vi "ReadDefaultConfig.vi"(8 "path":path, 11 "File":string) -> (0 "error out":errorcluster, 2 "path":path, 3 "config":T1={"Bead locations"=[{"X"=0, "Y"=0}], "ROI"=80, "Experiment base path"=path "", "Image output subdir"="images", "Output mode"=enum."Track", "Traces output subdir"="traces", "QTrk Settings"={"Image width"=100, "Image height"=100, "Number of threads (CPU based)"=-1, "CUDA Device"=-2, "COM Background correction factor"=0.0, "ZLUT MinRadius"=2.0, "ZLUT Radial sample density"=2.0, "ZLUT Angular sample density"=0.7, "ZLUT ROI Coverage"=1.0, "QI Iterations"=5, "QI MinRadius"=2.0, "QI Radial sample density"=2.0, "QI Angular sample density"=0.7, "QI ROI Coverage"=1.0, "QI Angular Step \nIteration Factor"=1.0, "XCOR Profile Length"=1, "XCOR Profile Width"=128, "XCOR Iterations"=32, "Gaussian 2D Fit Iterations"=2, "Gaussian 2D Sigma (pixels)"=3.0, "Downsample"=0}, "Tracking Config"={"Number of steps"=100, "ZLUT stepsize (um)"=0.05, "Z correction factor"=0.88, "Start piezo Z (um)"=0.0, "Pixel size (nm)"=146.0, "2D Localization Type"=enum."Quadrant Interpolation", "Z Command (None)"=enum."ComputeZ", "Z Piezo scale"=FALSE, "ZLUT Building\nimages per frame"=1, "ZLUT Bias correction planes"=1}, "Experiment Name"="test", "Program"={"Commands"=[], "Motor Axis accuracy conditions"={"Magnet Z"=0.0, "Magnet rotation"=0.0, "Camera"={"X"=0.0, "Y"=0.0}, "Piezo XY"={"X"=0.0, "Y"=0.0}, "Piezo Z"=0.0}, "Axis flags"={"Magnet Z"=FALSE, "Magnet rotation"=FALSE, "Camera"={"X"=FALSE, "Y"=FALSE}, "Piezo XY"={"X"=FALSE, "Y"=FALSE}, "Piezo Z"=FALSE}}, "ZLUT"=[], "Camera settings"={"Framerate (Hz)"=60, "Exposure time (us)"=5000, "Image size"={"Width"=1280, "Height"=1024}, "Number of buffers"=30}, "Experiment Script"="", "Max frames in memory"=100000, "Save traces as binary"=FALSE, "Pixel Calibration Gain Image"="camera_calib_gain.bin", "Pixel Calibration Offset Image"="camera_calib_offset.bin", "Use pixel calibration images"=FALSE, "Internal camera settings"="", "Trace write interval"=100, "ExperimentComment"=""} {"QTrk Settings"."QI ROI Coverage" format="%_2g"; "QTrk Settings"."QI MinRadius" format="%.2f"; "QTrk Settings"."QI Angular sample density" format="%.3f"; "QTrk Settings"."QI Radial sample density" format="%.2f"; "QTrk Settings"."ZLUT Radial sample density" format="%.2f"; "QTrk Settings"."ZLUT MinRadius" format="%.2f"})   [LabVIEW 2011]
uses:
  Main/Typedefs/MeasureConfigType.ctl
  Main/Typedefs/MeasureConfigOutputMode.ctl
  qtrk/QTrkLVBinding/QTrkSettings.ctl
  Main/Typedefs/TrackingConfigType.ctl
  qtrk/QTrkLVBinding/QTrkLocalizationType.ctl
  qtrk/QTrkLVBinding/QTrkZCommandType.ctl
  Main/ExperimentProgram/ExperimentProgramType.ctl
  Main/ExperimentProgram/ExProgCommandType.ctl
  Main/ExperimentProgram/ExProgCommandEnumType.ctl
  Main/Motors/MotorAxisEnum.ctl
  Main/Motors/MotorPosType.ctl
  Main/Typedefs/XYf.ctl
  Main/Motors/MotorPosFlagsType.ctl
  Main/Camera/GenericCameraConfigType.ctl
  Main/GlobalVariables.vi
  <vilib>/regexp/Match Regular Expression.xnode
panel:
  # "(used for commands with string parameters)"
  # "-2: Use all devices\n-1: Use best device"
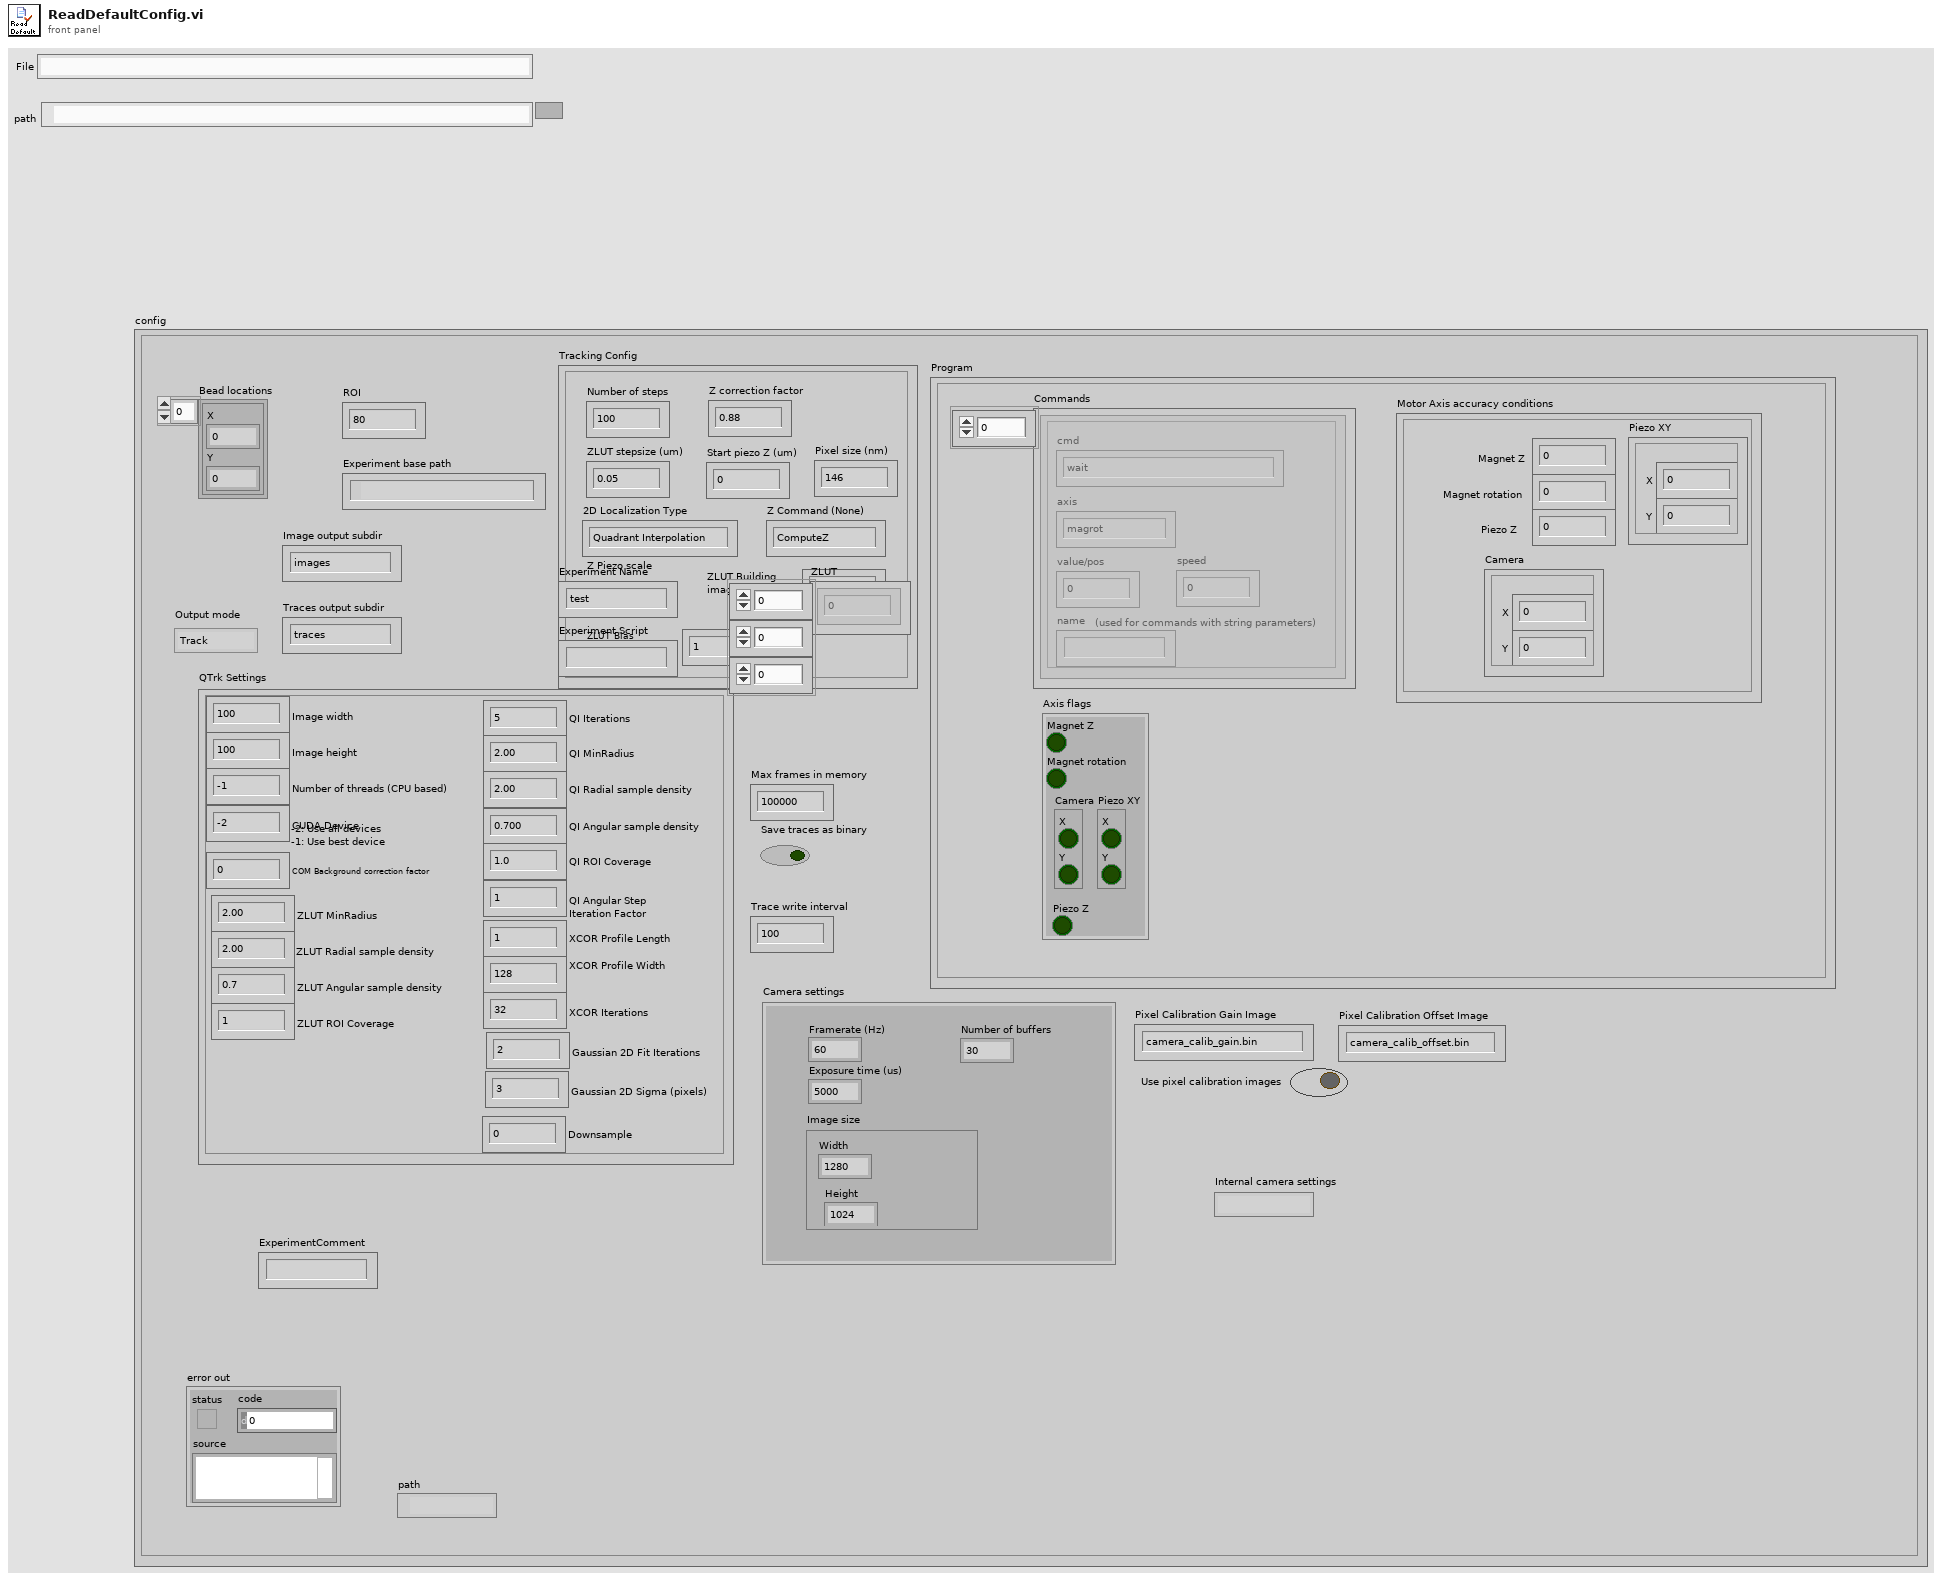
[diagram p1: front panel]
types:
  T1 = typedef "MeasureConfigType.ctl" = cluster{"Bead locations":cluster{"X":i32, "Y":i32}[], "ROI":i32, "Experiment base path":path, "Image output subdir":string, "Output mode":T2, "Traces output subdir":string, "QTrk Settings":T3, "Tracking Config":T4, "Experiment Name":string, "Program":T7, "ZLUT":sgl[][][], "Camera settings":T14, "Experiment Script":string, "Max frames in memory":i32, "Save traces as binary":bool, "Pixel Calibration Gain Image":string, "Pixel Calibration Offset Image":string, "Use pixel calibration images":bool, "Internal camera settings":string, "Trace write interval":i32, "ExperimentComment":string}
  T2 = typedef "MeasureConfigOutputMode.ctl" = enum16{"None", "Track", "SaveImages"}
  T3 = typedef "QTrkSettings.ctl" = cluster{"Image width":i32, "Image height":i32, "Number of threads (CPU based)":i32, "CUDA Device":i32, "COM Background correction factor":sgl, "ZLUT MinRadius":sgl, "ZLUT Radial sample density":sgl, "ZLUT Angular sample density":sgl, "ZLUT ROI Coverage":sgl, "QI Iterations":i32, "QI MinRadius":sgl, "QI Radial sample density":sgl, "QI Angular sample density":sgl, "QI ROI Coverage":sgl, "QI Angular Step \nIteration Factor":sgl, "XCOR Profile Length":i32, "XCOR Profile Width":i32, "XCOR Iterations":i32, "Gaussian 2D Fit Iterations":i32, "Gaussian 2D Sigma (pixels)":sgl, "Downsample":i32}
  T4 = typedef "TrackingConfigType.ctl" = cluster{"Number of steps":i32, "ZLUT stepsize (um)":sgl, "Z correction factor":sgl, "Start piezo Z (um)":sgl, "Pixel size (nm)":sgl, "2D Localization Type":T5, "Z Command (None)":T6, "Z Piezo scale":bool, "ZLUT Building\nimages per frame":i32, "ZLUT Bias correction planes":i32}
  T5 = typedef "QTrkLocalizationType.ctl" = enum16{"Center-of-Mass", "1D Cross-Correlation", "Quadrant Interpolation", "Gaussian 2D MLE", "QI + ZLUTAlign", "ZLUTAlign", "QI + FourierLUT"}
  T6 = typedef "QTrkZCommandType.ctl" = enum16{"Nothing", "ComputeZ", "BuildRadialZLUT", "BuildImageZLUT", "RadialZLUT+ImageZLUT"}
  T7 = typedef "ExperimentProgramType.ctl" = cluster{"Commands":T8[], "Motor Axis accuracy conditions":T11, "Axis flags":T13}
  T8 = typedef "ExProgCommandType.ctl" = cluster{"cmd":T9, "axis":T10, "value/pos":dbl, "speed":dbl, "name":string}
  T9 = typedef "ExProgCommandEnumType.ctl" = enum16{"wait", "move", "event", "idle", "when", "section", "stop"}
  T10 = typedef "MotorAxisEnum.ctl" = enum16{"no axis", "magrot", "magpos", "px", "py", "pz", "camx", "camy"}
  T11 = typedef "MotorPosType.ctl" = cluster{"Magnet Z":dbl, "Magnet rotation":dbl, "Camera":T12, "Piezo XY":T12, "Piezo Z":dbl}
  T12 = typedef "XYf.ctl" = cluster{"X":sgl, "Y":sgl}
  T13 = typedef "MotorPosFlagsType.ctl" = cluster{"Magnet Z":bool, "Magnet rotation":bool, "Camera":cluster{"X":bool, "Y":bool}, "Piezo XY":cluster{"X":bool, "Y":bool}, "Piezo Z":bool}
  T14 = typedef "GenericCameraConfigType.ctl" = cluster{"Framerate (Hz)":i32, "Exposure time (us)":i32, "Image size":cluster{"Width":i32, "Height":i32}, "Number of buffers":i32}
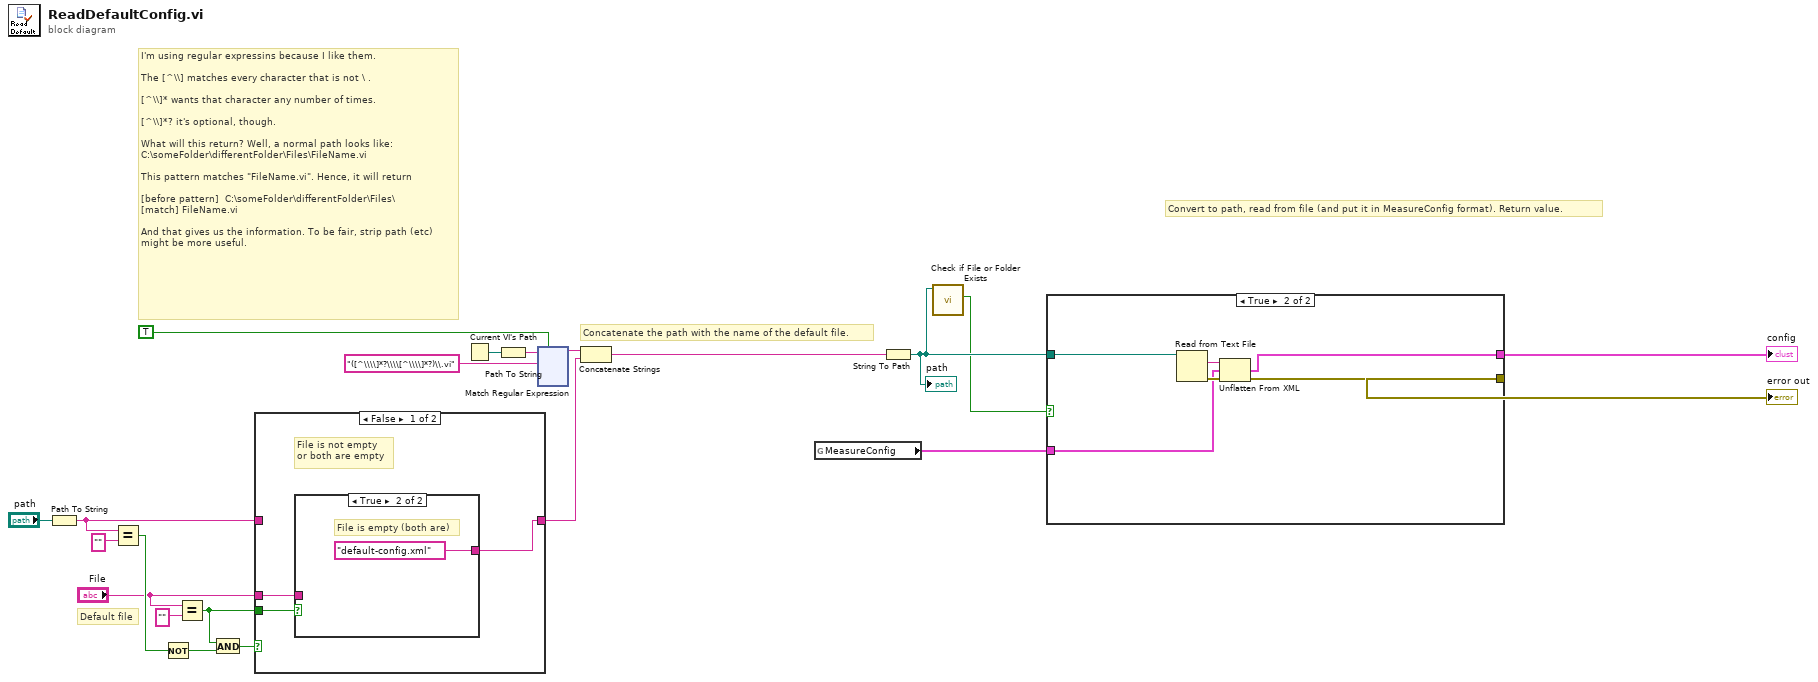
[diagram p0: block diagram]
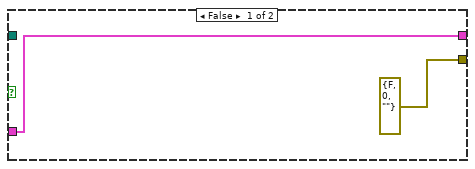
[diagram p2: hidden frame]
diagram:
  # "Convert to path, read from file (and put it in MeasureConfig format). Return value."
  # "Concatenate the path with the name of the default file."
  # "Default file"
  # "I'm using regular expressins because I like them. \n\nThe [^\\\\] matches every character that is not \\ . \n\n[^\\\\]* wants that character any number of times.\n\n[^\\\\]*? it's optional, though.\n\nWhat will this return? Well, a normal path looks like:\nC:\\someFolder\\differentFolder\\Files\\FileName.vi \n\nThis pattern matches \"FileName.vi\". Hence, it will return\n\n[before pattern]  C:\\someFolder\\differentFolder\\Files\\\n[match] FileName.vi\n\nAnd that gives us the information. To be fair, strip path (etc)\nmight be more useful."
  n1 = Path To String(path="path") -> (string=w5:string)
  n2 = Equal?(x=w5, y="") -> (x = y?=w8:bool)
  n3 = Not(x=w8) -> (.not. x?=w9:bool)
  n4 = Equal?(x="File", y="") -> (x = y?=w3:bool)
  n5 = And(x=w3, y=w9) -> (x .and. y?=w7:bool)
  n6 = case shown="False" w7 {
    tunnel: "File" -> [w22 _]
    tunnel: w5 -> [_ w27]
    tunnel: [w23 w27] -> w4
    tunnel: w3 -> [w24 _]
    frame False {
      # "File is not empty\nor both are empty"
      n7 = case shown="True" w24 {
        tunnel: [w25 "default-config.xml" ("File")] -> w23
        tunnel: w22 -> [w25 _]
        frame False {
          # "File is not empty"
        }
        frame True {
          # "File is empty (both are)"
        }
      }
    }
    frame True {
      # "File is empty, path is not"
    }
  }
  n8 = Current VI's Path() -> (path=w14:path)
  n9 = Path To String(path=w14) -> (string=w15:string)
  n10 = xnode "Match Regular Expression"("input string"=w15, "regular expression"="([^\\\\]*?\\\\[^\\\\]*?)\\.vi", "ignore case? (F)"=TRUE) -> ("before match"=w19:string)  [unwired: 3 in, 4 out]
  n11 = Concatenate Strings(w19, w4) -> (w20:string)
  n12 = global read "GlobalVariables.vi" "MeasureConfig"() -> (w18:T1)
  n13 = String To Path(string=w20) -> (path=w2:path)
  "path" <- w2
  n14 = call <vilib>:"Check if File or Folder Exists.vi"("path"=w2) -> ("file or folder exists?"=w1:bool)  [unwired: 8 in, 2 out]
  n15 = case shown="True" w1 {
    tunnel: [w29 w30] -> w21
    tunnel: w2 -> [_ w35]
    tunnel: w18 -> [w29 w31]
    tunnel: [errorcluster {"status"=FALSE, "code"=0, "source"=""} ("error out") w33] -> w13
    frame False {
    }
    frame True {
      n16 = Read from Text File(file (use dialog)=w35) -> (text=w34:string, error out=w32:errorcluster)  [unwired: 3 in, 2 out]
      n17 = Unflatten From XML(xml string=w34, type=w31, error in (no error)=w32) -> (value=w30:T1, error out=w33:errorcluster)
    }
  }
  "config" <- w21
  "error out" <- w13
